vi "Get Auton Steps.vi"(1 "Name of Auton to Do":string="left cargo") -> (0 "Output Movements":T1[](array[typedef]))   [LabVIEW 2018]
uses:
  Auton Movements.ctl
panel:
  in  "Auton Steps for Each AutonName":cluster{"Drive":dbl, "TurnDegrees":dbl}[][](array[cluster])=[[{"Drive"=73.35, "TurnDegrees"=-18.4}, {"Drive"=34.44, "TurnDegrees"=18.4}, {"Drive"=0.0, "TurnDegrees"=0.0}], [{"Drive"=73.35, "TurnDegrees"=18.4}, {"Drive"=34.44, "TurnDegrees"=-18.4}, {"Drive"=0.0, "TurnDegrees"=0.0}], [{"Drive"=48.24, "TurnDegrees"=27.0}, {"Drive"=172.551, "TurnDegrees"=-150.8}, {"Drive"=39.1, "TurnDegrees"=33.8}], [{"Drive"=48.24, "TurnDegrees"=27.0}, {"Drive"=172.551, "TurnDegrees"=-117.0}, {"Drive"=32.5, "TurnDegrees"=0.0}], [{"Drive"=48.24, "TurnDegrees"=27.0}, {"Drive"=172.551, "TurnDegrees"=-83.2}, {"Drive"=39.106, "TurnDegrees"=33.8}], [{"Drive"=48.24, "TurnDegrees"=-27.0}, {"Drive"=172.551, "TurnDegrees"=150.8}, {"Drive"=39.1, "TurnDegrees"=-33.8}], [{"Drive"=48.24, "TurnDegrees"=-27.0}, {"Drive"=172.551, "TurnDegrees"=117.0}, {"Drive"=32.5, "TurnDegrees"=0.0}], [{"Drive"=48.24, "TurnDegrees"=-27.0}, {"Drive"=172.551, "TurnDegrees"=83.2}, {"Drive"=39.106, "TurnDegrees"=-33.8}], [{"Drive"=48.24, "TurnDegrees"=-46.4}, {"Drive"=59.414, "TurnDegrees"=64.7}, {"Drive"=34.44, "TurnDegrees"=-18.4}], [{"Drive"=48.24, "TurnDegrees"=-46.4}, {"Drive"=59.414, "TurnDegrees"=28.0}, {"Drive"=34.44, "TurnDegrees"=18.4}], [{"Drive"=48.24, "TurnDegrees"=13.0}, {"Drive"=157.742, "TurnDegrees"=-136.8}, {"Drive"=39.106, "TurnDegrees"=33.8}], [{"Drive"=48.24, "TurnDegrees"=13.0}, {"Drive"=157.742, "TurnDegrees"=-103.0}, {"Drive"=32.5, "TurnDegrees"=0.0}], [{"Drive"=48.24, "TurnDegrees"=13.0}, {"Drive"=157.742, "TurnDegrees"=-69.2}, {"Drive"=39.106, "TurnDegrees"=-33.8}], [{"Drive"=48.24, "TurnDegrees"=46.4}, {"Drive"=59.414, "TurnDegrees"=-64.7}, {"Drive"=34.44, "TurnDegrees"=18.4}], [{"Drive"=48.24, "TurnDegrees"=46.4}, {"Drive"=59.414, "TurnDegrees"=-28.0}, {"Drive"=34.484, "TurnDegrees"=-18.4}], [{"Drive"=48.24, "TurnDegrees"=-13.0}, {"Drive"=157.742, "TurnDegrees"=136.8}, {"Drive"=39.106, "TurnDegrees"=-33.8}], [{"Drive"=48.24, "TurnDegrees"=-13.0}, {"Drive"=157.742, "TurnDegrees"=103.0}, {"Drive"=32.5, "TurnDegrees"=0.0}], [{"Drive"=48.24, "TurnDegrees"=-13.0}, {"Drive"=157.742, "TurnDegrees"=69.2}, {"Drive"=39.106, "TurnDegrees"=33.8}]]
  in  "AutonNames":string[](array[string])=["center -> fl", "center -> fr", "center -> r1", "center -> r2", "center -> r3", "center -> l1", "center -> l2", "center -> l3", "right -> fr", "right -> fl", "right -> r1", "right -> r2", "right -> r3", "left -> fl", "left -> fr", "left -> l1", "left -> l2", "left -> l3"]
  # "STUB VI"
  # "Needs appropriate values for each auton step"
  # "Counter-Clockwise is negative"
  # "Array of TypeDef Auton Movements"
  # "Left Cargo"
  # "Value of this up here needs to correspond\nto an AutonName"
  # "<---------\n# of rows = number of Auton Names\n# of columns = number of Auton Steps"
  # "The number of columns here need to \nbe equal to the number of Auton Steps"
  # "This essentially acts as a bank to pull the\nsteps from once they are found"
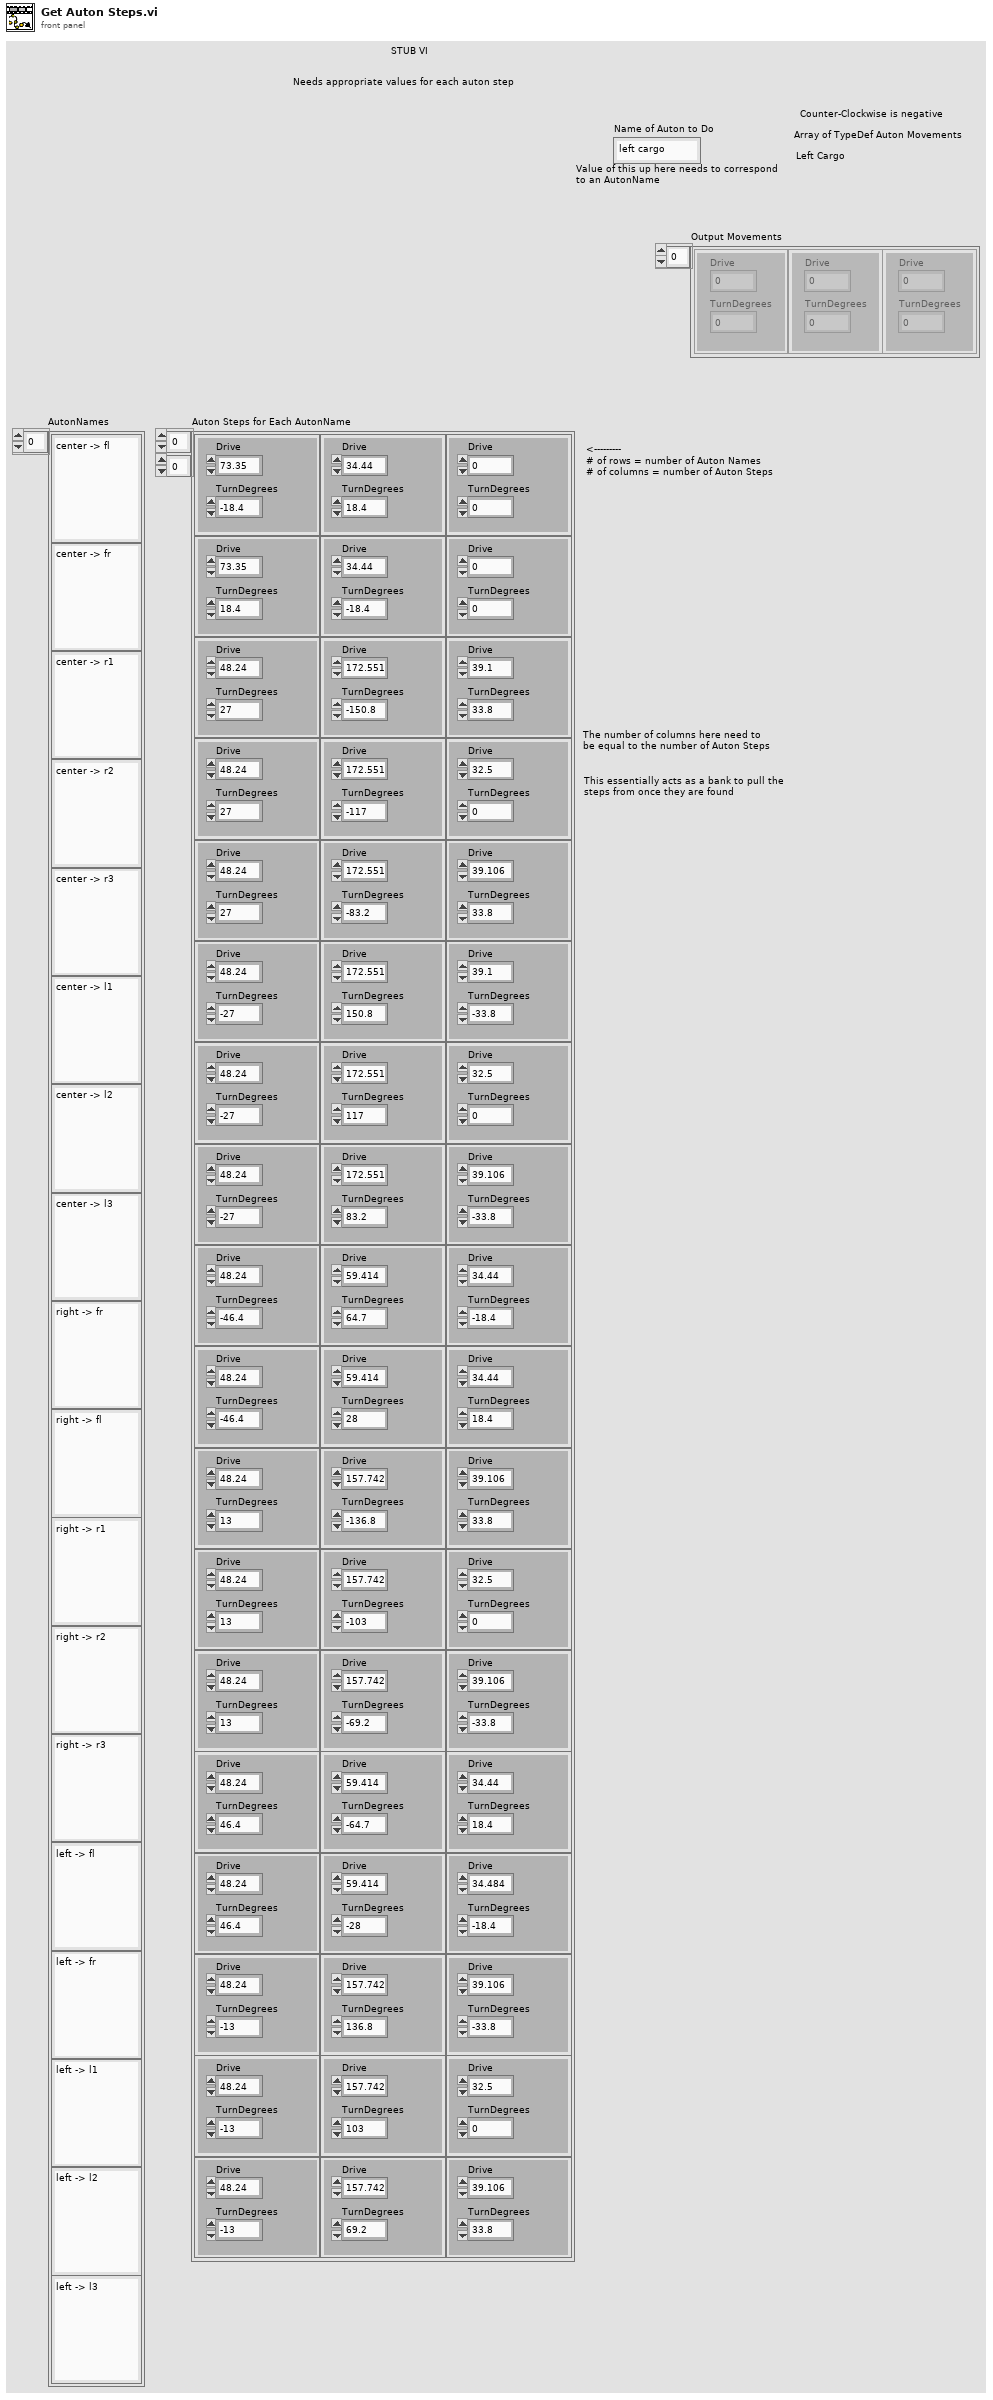
[diagram p1: front panel]
types:
  T1 = typedef "Auton Movements.ctl" = cluster{"Drive":dbl, "TurnDegrees":dbl}
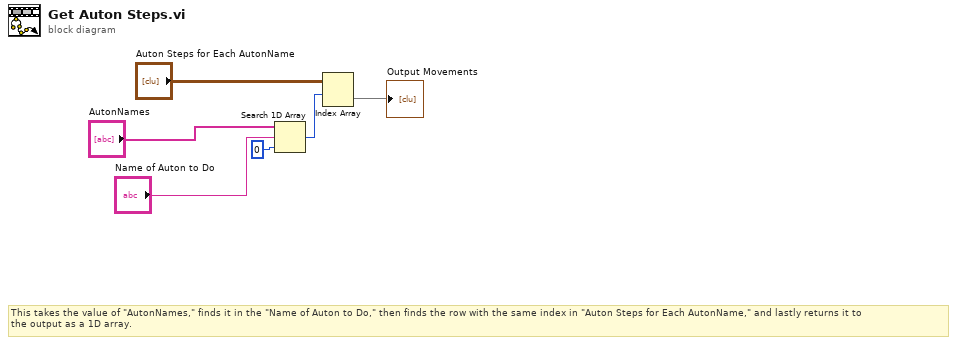
[diagram p0: block diagram]
diagram:
  # "This takes the value of \"AutonNames,\" finds it in the \"Name of Auton to Do,\" then finds the row with the same index in \"Auton Steps for Each AutonName,\" and lastly returns it to\nthe output as a 1D array."
  n1 = Search 1D Array(1D array="AutonNames", element="Name of Auton to Do", start index (0)=0) -> (index of element=w2:i32)
  n2 = Index Array(array="Auton Steps for Each AutonName", index (row)=w2) -> (element=→"Output Movements":cluster{"Drive":dbl, "TurnDegrees":dbl}[])  [unwired: 1 in]
